vi "Exchange-element.vi"(8 "error in (no error)":errorcluster, 10 "Element-XML in 2":refnum<class "Element-XML.lvclass">, 11 "Element-XML in":refnum<class "Element-XML.lvclass">) -> (0 "error out":errorcluster, 2 "Element-XML out 2":refnum<class "Element-XML.lvclass">, 3 "Element-XML out":refnum<class "Element-XML.lvclass">)   [LabVIEW 2013, in "HardwareCharacterization.lvlib" / "Element-XML.lvclass"]
uses:
  Element-XML.lvclass
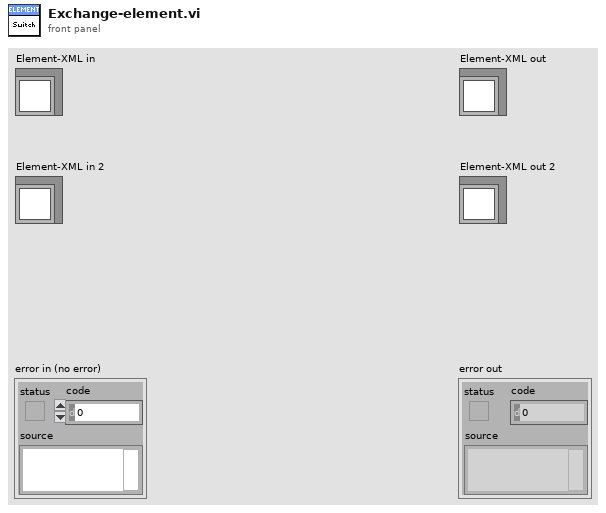
[diagram p1: front panel]
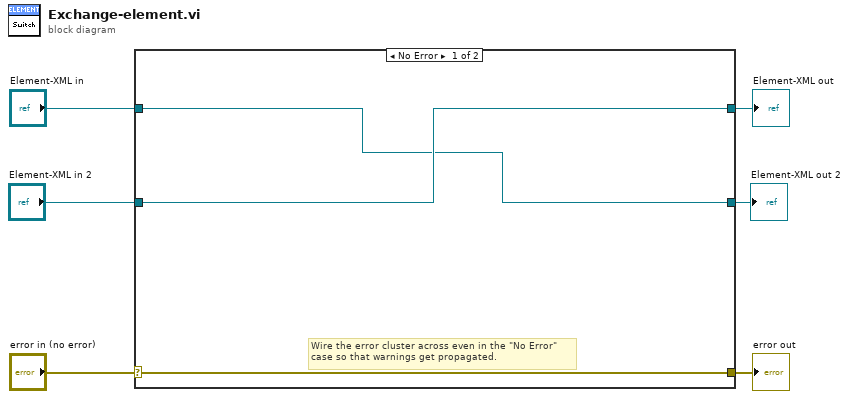
[diagram p0: block diagram]
diagram:
  n1 = case shown="No Error" "error in (no error)" {
    selector: "error in (no error)" -> [w9 w12]
    tunnel: [w9 w12] -> w5
    tunnel: [w8 w11] -> w3
    tunnel: "Element-XML in" -> [w7 w11]
    tunnel: "Element-XML in 2" -> [w8 w10]
    tunnel: [w7 w10] -> w1
    frame No Error {
      # "Wire the error cluster across even in the \"No Error\"\ncase so that warnings get propagated."
    }
    frame Error {
    }
  }
  "error out" <- w5
  "Element-XML out" <- w3
  "Element-XML out 2" <- w1
